vi "Ejercicio_8_String_Concatenar.vi"() -> ()   [LabVIEW 2020]
panel:
  out "output 1":dbl
  out "before substring":string
  out "after substring":string
  out "match substring":string
  out "offset past match":i32
  in  "input 1":dbl
  out "Longitud":i32
  in  "Unidades":string
  in  "Encabezado":string="El valor del voltaje es:"
  out "concatenated string":string
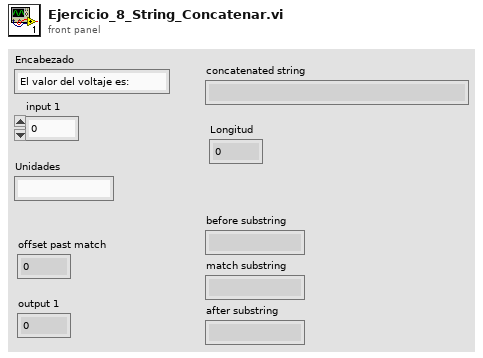
[diagram p1: front panel]
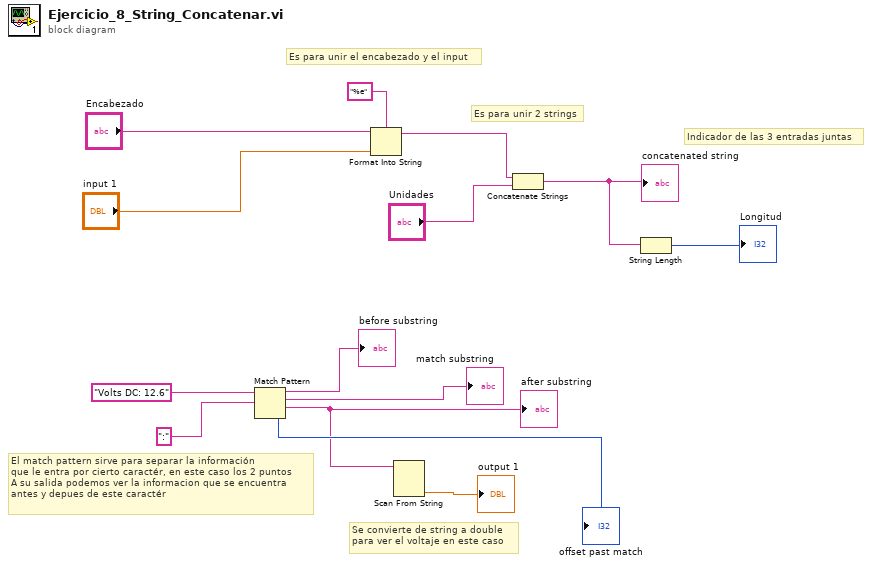
[diagram p0: block diagram]
diagram:
  # "Indicador de las 3 entradas juntas"
  # "Es para unir 2 strings"
  # "Es para unir el encabezado y el input"
  # "Se convierte de string a double \npara ver el voltaje en este caso"
  # "El match pattern sirve para separar la información\nque le entra por cierto caractér, en este caso los 2 puntos\nA su salida podemos ver la informacion que se encuentra\nantes y depues de este caractér"
  n1 = Match Pattern(string="Volts DC: 12.6", regular expression=":") -> (before substring=→"before substring":string, match substring=→"match substring":string, after substring=w1:string, offset past match=→"offset past match":i32)  [unwired: 1 in]
  "after substring" <- w1
  n2 = Format Into String "Format Into String"(format string="%e", initial string="Encabezado", "input 1") -> (resulting string=w13:string)  [unwired: 1 in, 1 out]
  n3 = Scan From String "Scan From String"(input string=w1) -> (output 1=→"output 1":dbl)  [unwired: 4 in, 3 out]
  n4 = Concatenate Strings "Concatenate Strings"(w13, "Unidades") -> (w12:string)
  "concatenated string" <- w12
  n5 = String Length(string=w12) -> (length=→"Longitud":i32)
